vi "Hologram.vi"() -> ()   [LabVIEW 2016]
uses:
  <vilib>/Math Plots/3D Math Plots/3D Surface/3D Surface XCtrl/3D Surface.xctl
  <vilib>/Analysis/2dsp.llb/2D Real FFT.vi
  <vilib>/Analysis/2dsp.llb/2D Inverse Complex FFT.vi
  <vilib>/gmath/interp.llb/Create Mesh Grid (2D) (x,y arrays).vi
  <vilib>/Math Plots/3D Math Plots/3D Surface/3D Surface Datatype/Public/Plot Helper (Matrix).vi
  <vilib>/imath/engines/lvmath2/RunTimeEngine/Managers/WorkSpace/UID Generator.vi
  <vilib>/imath/engines/lvmath2/RunTimeEngine/RunTimeType/NIMS_RunTimeType_From StrictType (excl LVString).vi
  <instcachedir>/0/NIMS_RunTimeType_From StrictType (excl LVString)_CEE1C65A8F1B491DB327E5E54E5E7674.lvgen/NIMS_RunTimeType_From StrictType (excl LVString)_CEE1C65A8F1B491DB327E5E54E5E7674_000.vi
  <vilib>/imath/engines/lvmath2/RunTimeEngine/LocalVariableDefStatement/MC_LocalVariableDefStatement_Display.vi
  <vilib>/imath/engines/lvmath2/RunTimeEngine/RangeToken/NIMS_Range.vi
  <instcachedir>/0/NIMS_Range_B290C9A4B417448F8AD7612DC5651788.lvgen/NIMS_Range_B290C9A4B417448F8AD7612DC5651788_001.vi
  <vilib>/imathl/engines/lvmath/Functions/Error Handling/Create Error.vi
  <vilib>/imath/engines/lvmath2/RunTimeEngine/IndexReplace/NIMS M(V,V)=S.vi
  <instcachedir>/0/NIMS M(V,V)=S_B76AA88630A24ACABE42EB78AC5194F0.lvgen/NIMS M(V,V)=S_B76AA88630A24ACABE42EB78AC5194F0_000.vi
  <vilib>/imath/engines/lvmath2/RunTimeEngine/ArithmeticOperatorToken/NIMS_ArithmeticOperator_times.vi
  <instcachedir>/0/NIMS_ArithmeticOperator_times_29A23DE60350445AA3495882984401F9.lvgen/NIMS_ArithmeticOperator_times_29A23DE60350445AA3495882984401F9_009.vi
  <vilib>/imath/engines/lvmath2/RunTimeEngine/BuiltInFunctions/circularshift/NIMS_circularshift(GM,V).vi
  <instcachedir>/0/NIMS_circularshift(GM,V)_7F2A11F2611744A7BE142894898AB4A4.lvgen/NIMS_circularshift(GM,V)_7F2A11F2611744A7BE142894898AB4A4_000.vi
  <vilib>/imath/engines/lvmath2/RunTimeEngine/Managers/SymbolTable/Clear UID.vi
  <vilib>/imath/engines/lvmath2/RunTimeEngine/NodeEndStatement/NIMS_NodeEndStatement_Output.vi
  <instcachedir>/0/NIMS_NodeEndStatement_Output_53EC0D466D134D7ABD903AC30B43404B.lvgen/NIMS_NodeEndStatement_Output_53EC0D466D134D7ABD903AC30B43404B_003.vi
  <vilib>/imath/engines/lvmath2/RunTimeEngine/ErrorHandling/NIMS_Finalize Error.vi
  <vilib>/imath/engines/lvmath2/RunTimeEngine/ArithmeticOperatorToken/NIMS_ArithmeticOperator_plus.vi
  <instcachedir>/0/NIMS_ArithmeticOperator_plus_C66E168CFD7E4B8EADE9B07A37DF7C62.lvgen/NIMS_ArithmeticOperator_plus_C66E168CFD7E4B8EADE9B07A37DF7C62_003.vi
  <vilib>/imath/engines/lvmath2/RunTimeEngine/ArithmeticOperatorToken/NIMS_ArithmeticOperator_power(S).vi
  <instcachedir>/0/NIMS_ArithmeticOperator_power(S)_EC726B27903B43E7ADD85D84A4E4D408.lvgen/NIMS_ArithmeticOperator_power(S)_EC726B27903B43E7ADD85D84A4E4D408_014.vi
  <instcachedir>/0/NIMS_NodeEndStatement_Output_53EC0D466D134D7ABD903AC30B43404B.lvgen/NIMS_NodeEndStatement_Output_53EC0D466D134D7ABD903AC30B43404B_002.vi
  <vilib>/Math Plots/3D Math Plots/3D Surface/3D Surface Datatype/3D Surface Datatype.lvclass
  <vilib>/gmath/NI_Gmath.lvlib
  <vilib>/Analysis/NI_AALPro.lvlib
  <vilib>/imath/engines/lvmath2/RunTimeEngine/Managers/SymbolTable/NIMS_WorkSpace.lvlib
panel:
  in  "Path":path
  out "fihnew":dbl[][](array[numeric])
  out "Array 6":dbl[][](array[numeric])
  out "angle(ifft)":picture
  out "abs ifft":refnum<class "3D Plot Datatype.lvclass">[](xcontrol)
  out "ifft of Mask":picture
  out "Array 2":cdb[][](array[numeric])
  out "Array":dbl[][](array[numeric])
  out "Mask":picture
  out "log Fih":dbl[][](array[numeric])
  out "pt 2":cdb[][](array[numeric]) format="%#_1g"
  out "KX  + KY":cdb[][](array[numeric])
  out "KY":dbl[][](array[numeric])
  out "KX":dbl[][](array[numeric])
  out "ref wave raw":cdb[][](array[numeric]) format="%#_2g"
  out "Hologram":dbl[][](array[numeric])
  out "ref wave u8":dbl[][](array[numeric])
  out "IH":dbl[][](array[numeric])
  out "255*H/max":dbl[][](array[numeric])
  out "H/max":dbl[][](array[numeric])
  out "Max value":dbl format="%#_5g"
  out "Objwave":dbl[][](array[numeric])
  out "Fourier Space":picture
  out "Fih":picture
  out "FIH":dbl[][](array[numeric])
  out "Hologram":picture
  out "Reference Wave":picture
  out "Object Wave":picture
  out "Original Image 2":refnum<class "3D Plot Datatype.lvclass">[](xcontrol)
  out "Original Image":refnum<class "3D Plot Datatype.lvclass">[](xcontrol)
  # "FIh"
  # "Image"
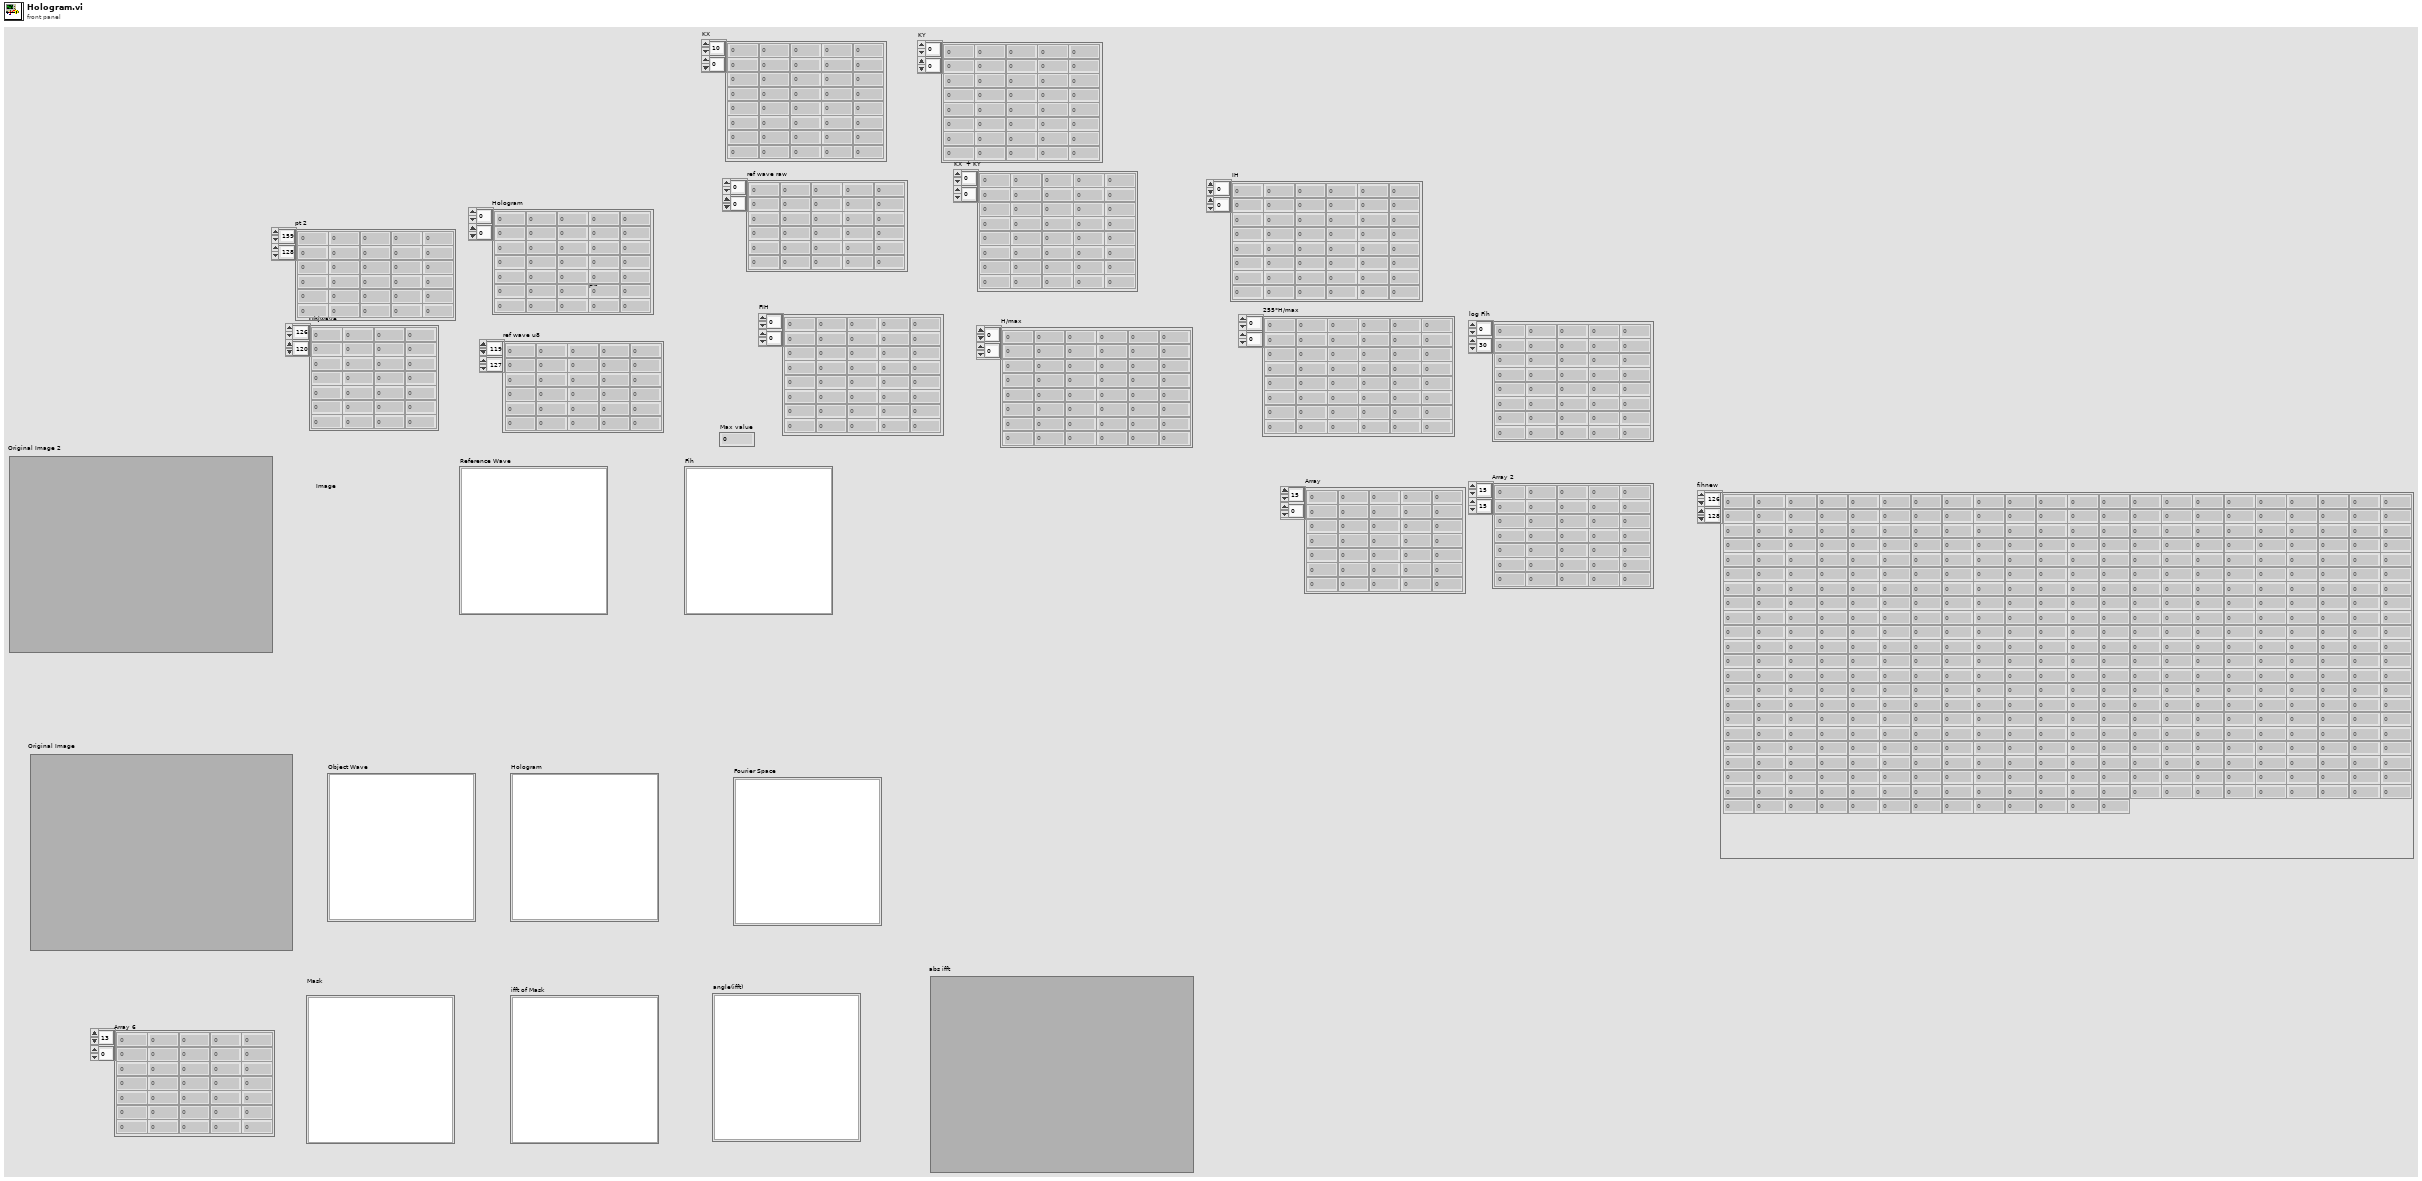
[diagram p1: front panel]
types:
  T1 = typedef "imagedata.ctl" = cluster{"image type":i32, "image depth":i32, "image":u8[], "mask":u8[], "colors":u32[], "Rectangle":cluster{"left":i16, "top":i16, "right":i16, "bottom":i16}}
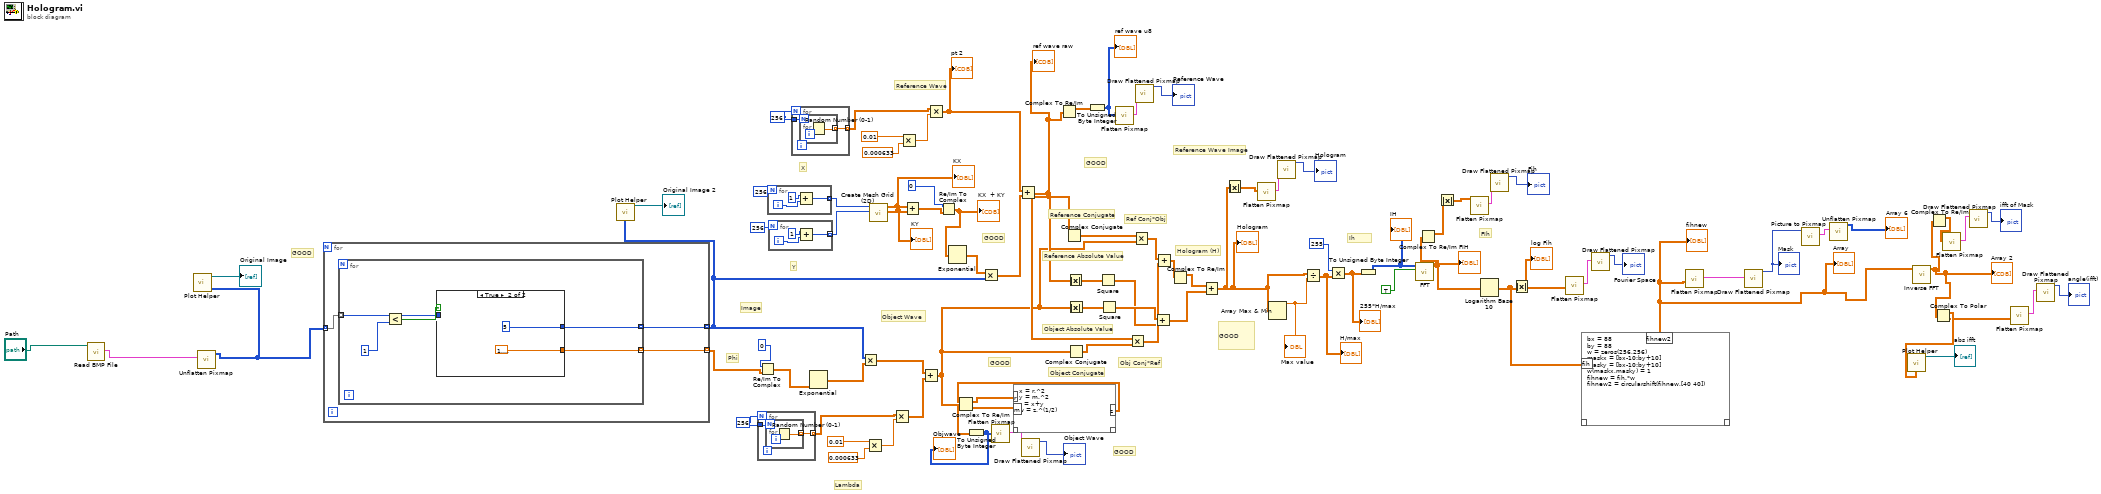
[diagram p0: block diagram]
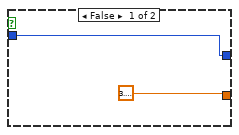
[diagram p2: hidden frame]
diagram:
  w76 = 256
  w88 = 256
  # "Phi"
  # "Image"
  # "GOOD"
  # "GOOD"
  # "GOOD"
  # "GOOD"
  # "GOOD"
  # "GOOD"
  # "FIh"
  # "Ih"
  # "Hologram (H)"
  # "Ref Conj*Obj"
  # "Obj Conj*Ref"
  # "Reference Conjugate"
  # "Reference Absolute Value"
  # "Object Absolute Value"
  # "Object Conjugate"
  # "Reference Wave Image"
  # "Y"
  # "X"
  # "Lambda"
  # "Reference Wave"
  # "Object Wave"
  n1 = call <vilib>:"Read BMP File.vi"("path to BMP file"="Path") -> ("image data"=w50:T1)  [unwired: 8 in, 2 out]
  n2 = call <vilib>:"Unflatten Pixmap.vi"("image data"=w50) -> ("24-bit pixmap"=w6:u32[][])  [unwired: 4 in, 6 out]
  n3 = call-poly <vilib>:"Plot Helper.vi"("z matrix"=w6) -> ("3D Plot lvclass Array out"=→"Original Image":refnum<class "3D Plot Datatype.lvclass">[])  [unwired: 5 in, 5 out]
  n4 = for {
    tunnel: w6 -> [w93] mode=indexing
    tunnel: [w92] -> w5 mode=indexing
    tunnel: [w91] -> w46 mode=indexing
    n5 = for {
      tunnel: w93 -> [w95] mode=indexing
      tunnel: [w94] -> w92 mode=indexing
      tunnel: [w96] -> w91 mode=indexing
      n6 = Less?(x=w95, y=1) -> (x < y?=w98:bool)
      n7 = case shown="True" w98 {
        tunnel: [w99 u32 5] -> w94
        tunnel: [3.141592653589793 1.5707963267948966] -> w96
        tunnel: w95 -> [w99 _]
        frame False {
        }
        frame True {
        }
      }
    }
  }
  n8 = call-poly <vilib>:"Plot Helper.vi"("z matrix"=w5) -> ("3D Plot lvclass Array out"=→"Original Image 2":refnum<class "3D Plot Datatype.lvclass">[])  [unwired: 5 in, 5 out]
  n9 = for {
    N: w88 -> [_]
    tunnel: w88 -> [w104]
    tunnel: [w103] -> w85 mode=indexing
    n10 = for {
      N: w104 -> [_]
      tunnel: [w105] -> w103 mode=indexing
      n11 = Random Number (0-1)() -> (number: 0 to 1=w105:dbl)
    }
  }
  n12 = Re/Im To Complex(1:w46, 2:0) -> (0:w45:cdb[][])
  n13 = for {
    N: 256 -> [_]
    tunnel: [w106] -> w69 mode=indexing
    i -> [w107]
    n14 = Add(x=1, y=w107) -> (x+y=w106:i32)
  }
  n15 = for {
    N: 256 -> [_]
    tunnel: [w109] -> w77 mode=indexing
    i -> [w110]
    n16 = Add(x=1, y=w110) -> (x+y=w109:i32)
  }
  n17 = for {
    N: w76 -> [_]
    tunnel: w76 -> [w113]
    tunnel: [w112] -> w70 mode=indexing
    n18 = for {
      N: w113 -> [_]
      tunnel: [w114] -> w112 mode=indexing
      n19 = Random Number (0-1)() -> (number: 0 to 1=w114:dbl)
    }
  }
  n20 = Exponential(1:w45) -> (0:w47:cdb[][])
  n21 = Multiply(x=w5, y=w47) -> (x*y=w83:cdb[][])
  n22 = Multiply(x=0.01, y=0.000633) -> (x*y=w84:dbl)
  n23 = call-poly <vilib>:"Create Mesh Grid (2D).vi"("y domain"=w77, "x domain"=w69) -> ("Y"=w42:dbl[][], "X"=w43:dbl[][])  [unwired: 7 in, 1 out]
  "KX" <- w43
  "KY" <- w42
  n24 = Multiply(x=w85, y=w84) -> (x*y=w82:dbl[][])
  n25 = Multiply(x=0.01, y=0.000633) -> (x*y=w73:dbl)
  n26 = Add(x=w43, y=w42) -> (x+y=w40:dbl[][])
  n27 = Add(x=w83, y=w82) -> (x+y=w32:cdb[][])
  n28 = Multiply(x=w70, y=w73) -> (x*y=w36:dbl[][])
  "pt 2" <- w36
  n29 = Re/Im To Complex(1:w40, 2:0) -> (0:w39:cdb[][])
  "KX  + KY" <- w39
  n30 = Exponential(1:w39) -> (0:w38:cdb[][])
  n31 = Complex To Re/Im(x + iy=w32) -> (x=w3:dbl[][], y=w2:dbl[][])
  n32 = Multiply(x=w38, y=w5) -> (x*y=w37:cdb[][])
  n33 = mathscript code="x = r.^2\ny = m.^2\nz = x+y\nw = z.^(1/2)"("r"=w3, "m"=w2) -> ("z"=w1:dbl[][])  [unwired: 1 in, 1 out]
  n34 = To Unsigned Byte Integer(number=w1) -> (unsigned 8bit integer=w26:u8[][])
  "Objwave" <- w26
  n35 = call <vilib>:"Flatten Pixmap.vi"("8-bit pixmap"=w26) -> ("image data"=w81:T1)  [unwired: 10 in]
  n36 = Add(x=w36, y=w37) -> (x+y=w34:cdb[][])
  "ref wave raw" <- w34
  n37 = call <vilib>:"Draw Flattened Pixmap.vi"("image data"=w81) -> ("new picture"=→"Object Wave":picture)  [unwired: 8 in]
  n38 = Complex To Re/Im(x + iy=w34) -> (x=w35:dbl[][])  [unwired: 1 out]
  n39 = Complex Conjugate(1:w34) -> (0:w51:cdb[][])
  n40 = Absolute Value(x=w34) -> (abs(x)=w67:dbl[][])
  n41 = Absolute Value(x=w32) -> (abs(x)=w68:dbl[][])
  n42 = Complex Conjugate(1:w32) -> (0:w66:cdb[][])
  n43 = To Unsigned Byte Integer(number=w35) -> (unsigned 8bit integer=w33:u8[][])
  "ref wave u8" <- w33
  n44 = Square(x=w67) -> (x^2=w62:dbl[][])
  n45 = Square(x=w68) -> (x^2=w65:dbl[][])
  n46 = call <vilib>:"Flatten Pixmap.vi"("8-bit pixmap"=w33) -> ("image data"=w72:T1)  [unwired: 10 in]
  n47 = Multiply(x=w34, y=w66) -> (x*y=w63:cdb[][])
  n48 = Multiply(x=w51, y=w32) -> (x*y=w64:cdb[][])
  n49 = call <vilib>:"Draw Flattened Pixmap.vi"("image data"=w72) -> ("new picture"=→"Reference Wave":picture)  [unwired: 8 in]
  n50 = Add(x=w65, y=w62) -> (x+y=w54:dbl[][])
  n51 = Add(x=w64, y=w63) -> (x+y=w53:cdb[][])
  n52 = Complex To Re/Im(x + iy=w53) -> (x=w52:dbl[][])  [unwired: 1 out]
  n53 = Add(x=w52, y=w54) -> (x+y=w31:dbl[][])
  "Hologram" <- w31
  n54 = Absolute Value(x=w31) -> (abs(x)=w27:dbl[][])
  n55 = call <vilib>:"Flatten Pixmap.vi"("8-bit pixmap"=w27) -> ("image data"=w60:T1)  [unwired: 10 in]
  n56 = Array Max & Min(array=w31) -> (max value=w30:dbl)  [unwired: 3 out]
  "Max value" <- w30
  n57 = call <vilib>:"Draw Flattened Pixmap.vi"("image data"=w60) -> ("new picture"=→"Hologram":picture)  [unwired: 8 in]
  n58 = Divide(x=w31, y=w30) -> (x/y=w49:dbl[][])
  "H/max" <- w49
  n59 = Multiply(x=255, y=w49) -> (x*y=w48:dbl[][])
  "255*H/max" <- w48
  n60 = To Unsigned Byte Integer(number=w48) -> (unsigned 8bit integer=w29:u8[][])
  "IH" <- w29
  n61 = call-poly <vilib>:"FFT.vi"("shift?"=TRUE, "X"=w29) -> ("FFT {X}"=w28:cdb[][])  [unwired: 8 in, 1 out]
  "FIH" <- w28
  n62 = Complex To Re/Im(x + iy=w28) -> (x=w56:dbl[][])  [unwired: 1 out]
  n63 = Absolute Value(x=w56) -> (abs(x)=w55:dbl[][])
  n64 = call <vilib>:"Flatten Pixmap.vi"("24-bit pixmap"=w55) -> ("image data"=w58:T1)  [unwired: 10 in]
  n65 = Logarithm Base 10(1:w28) -> (0:w10:cdb[][])
  n66 = call <vilib>:"Draw Flattened Pixmap.vi"("image data"=w58) -> ("new picture"=→"Fih":picture)  [unwired: 8 in]
  n67 = Absolute Value(x=w10) -> (abs(x)=w12:dbl[][])
  "log Fih" <- w12
  n68 = call <vilib>:"Flatten Pixmap.vi"("4-bit pixmap"=w12) -> ("image data"=w25:T1)  [unwired: 10 in]
  n69 = mathscript code="bx = 88\nby = 88\nw = zeros(256,256)\nmaskx = [bx-10:by+10]\nmasky = [bx-10:by+10]\nw(maskx,masky) = 1\nfihnew = fih.*w\nfihnew2 = circularshift(fihnew,[40 40])"("fih"=w10) -> ("fihnew2"=w9:cdb[][])  [unwired: 1 in, 1 out]
  "Array" <- w9
  "fihnew" <- w9
  n70 = call <vilib>:"Draw Flattened Pixmap.vi"("image data"=w25) -> ("new picture"=→"Fourier Space":picture)  [unwired: 8 in]
  n71 = call <vilib>:"Flatten Pixmap.vi"("4-bit pixmap"=w9) -> ("image data"=w11:T1)  [unwired: 10 in]
  n72 = call <vilib>:"Draw Flattened Pixmap.vi"("image data"=w11) -> ("new picture"=w15:picture)  [unwired: 8 in]
  "Mask" <- w15
  n73 = call <vilib>:"Picture to Pixmap.vi"("picture"=w15) -> ("image data"=w14:T1)  [unwired: 9 in, 1 out]
  n74 = call <vilib>:"Unflatten Pixmap.vi"("image data"=w14) -> ("24-bit pixmap"=→"Array 6":u32[][])  [unwired: 4 in, 6 out]
  n75 = call-poly <vilib>:"Inverse FFT.vi"("FFT {x}"=w9) -> ("X"=w8:cdb[][])  [unwired: 9 in, 1 out]
  "Array 2" <- w8
  n76 = Complex To Re/Im(x + iy=w8) -> (x=w7:dbl[][])  [unwired: 1 out]
  n77 = Complex To Polar(r * e^(i*theta)=w8) -> (r=w19:dbl[][], theta=w16:dbl[][])
  n78 = call-poly <vilib>:"Plot Helper.vi"("z matrix"=w19) -> ("3D Plot lvclass Array out"=→"abs ifft":refnum<class "3D Plot Datatype.lvclass">[])  [unwired: 5 in, 5 out]
  n79 = call <vilib>:"Flatten Pixmap.vi"("8-bit pixmap"=w7) -> ("image data"=w22:T1)  [unwired: 10 in]
  n80 = call <vilib>:"Draw Flattened Pixmap.vi"("image data"=w22) -> ("new picture"=→"ifft of Mask":picture)  [unwired: 8 in]
  n81 = call <vilib>:"Flatten Pixmap.vi"("4-bit pixmap"=w16) -> ("image data"=w18:T1)  [unwired: 10 in]
  n82 = call <vilib>:"Draw Flattened Pixmap.vi"("image data"=w18) -> ("new picture"=→"angle(ifft)":picture)  [unwired: 8 in]
